vi "Build HTML Response.vi"(9 "HTML":string="<html>\n     <body>\n            response here\n     </body>\n</html>", 10 "Status":string(combo)="200 OK", 11 "HTTP Version":string="HTTP/1.1") -> (3 "HTTP Response":string)   [LabVIEW 2020]
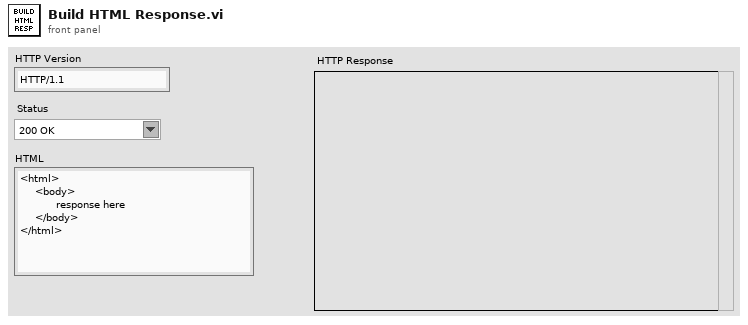
[diagram p1: front panel]
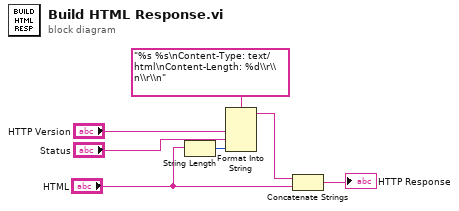
[diagram p0: block diagram]
diagram:
  n1 = String Length(string="HTML") -> (length=w4:i32)
  n2 = Format Into String(format string="%s %s\nContent-Type: text/html\nContent-Length: %d\\r\\n\\r\\n" ("regular expression"), "HTTP Version", "Status", w4) -> (resulting string=w2:string)  [unwired: 2 in, 1 out]
  n3 = Concatenate Strings(w2, "HTML") -> (→"HTTP Response":string)
